vi "CanRxDetector.vi"() -> ()   [LabVIEW 2012]
panel:
  out "string":string
  in  "CAN_ID_Filter":u32 format="%08x"
  out "Picture":picture
  out "is active":bool
  out "error out":errorcluster {"code" format="%.0x"}
  out "Channel Status":T1 {"TX Load (%)" max=100 scale=0.0..100.0; "RX Load (%)" max=100 scale=0.0..100.0; "Line Status"."BUS Timing"."BTR1" format="%02x"; "Line Status"."BUS Timing"."BTR0" format="%02x"; "Line Status"."BUS Load (%)" max=100 step=1 scale=0.0..100.0}
  in  "Stop":bool
  out "Message Count":u32
  out "CAN message":T2 {"Data"."[4]" format="%02x"; "Data"."[7]" format="%02x"; "Data"."[6]" format="%02x"; "Data"."[5]" format="%02x"; "Data"."[3]" format="%02x"; "Data"."[2]" format="%02x"; "Data"."[1]" format="%02x"; "Data"."[0]" format="%02x"; "Timestamp" format="%08x"; "Arbitration ID" format="%08x"}
  out "IsRunning":bool
  # "CAN messages Log"
  # "CAN ID"
  # "CAN message"
  # "Channel Status"
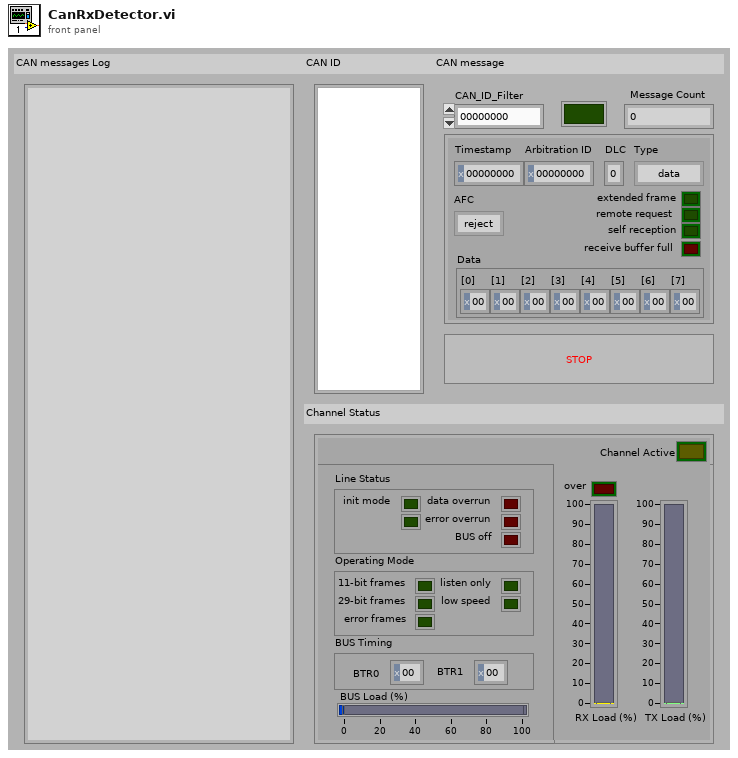
[diagram p1: front panel]
types:
  T1 = cluster{"Line Status":cluster{"Line Status":cluster{"init mode":bool, "TX pending":bool, "data overrun":bool, "error overrun":bool, "BUS off":bool}, "Operating Mode":cluster{"11-bit frames":bool, "29-bit frames":bool, "error frames":bool, "listen only":bool, "low speed":bool}, "BUS Timing":cluster{"BTR0":u8, "BTR1":u8}, "BUS Load (%)":u8}, "Channel Active":bool, "over":bool, "RX Load (%)":u8, "TX Load (%)":u8}
  T2 = cluster{"Timestamp":u32, "Arbitration ID":u32, "DLC":u8, "Type":enum8{"data", "info", "error", "status", "wakeup", "timer ovr", "timer reset"}, "AFC":enum8{"reject", "always", "filter 1", "filter 2"}, "extended frame":bool, "remote request":bool, "self reception":bool, "receive buffer full":bool, "Data":cluster{"[0]":u8, "[1]":u8, "[2]":u8, "[3]":u8, "[4]":u8, "[5]":u8, "[6]":u8, "[7]":u8}}
  T3 = cluster{"Width":u16, "Style":enum32{"Solid", "Dash", "Dot", "DashDot", "DashDotDot"}}
  T4 = cluster{"[0]":u8, "[1]":u8, "[2]":u8, "[3]":u8, "[4]":u8, "[5]":u8, "[6]":u8, "[7]":u8}
  T5 = cluster{"Data[0]":u8, "Data[1]":u8, "Data[2]":u8, "Data[3]":u8, "Data[4]":u8, "Data[5]":u8, "Data[6]":u8, "Data[7]":u8}
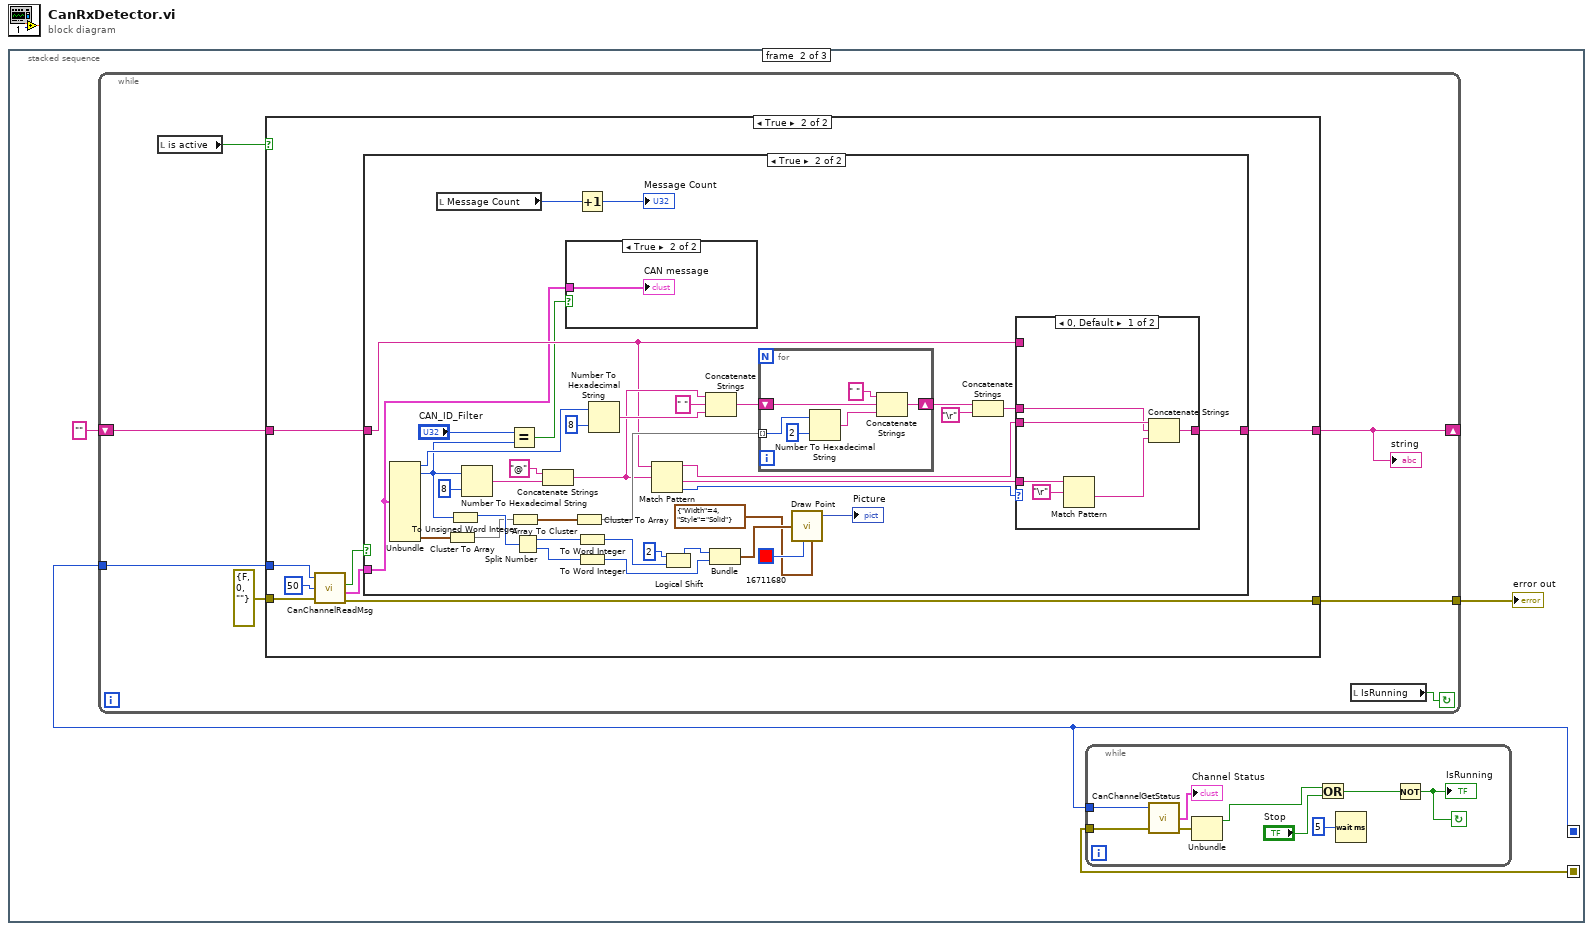
[diagram p0: block diagram]
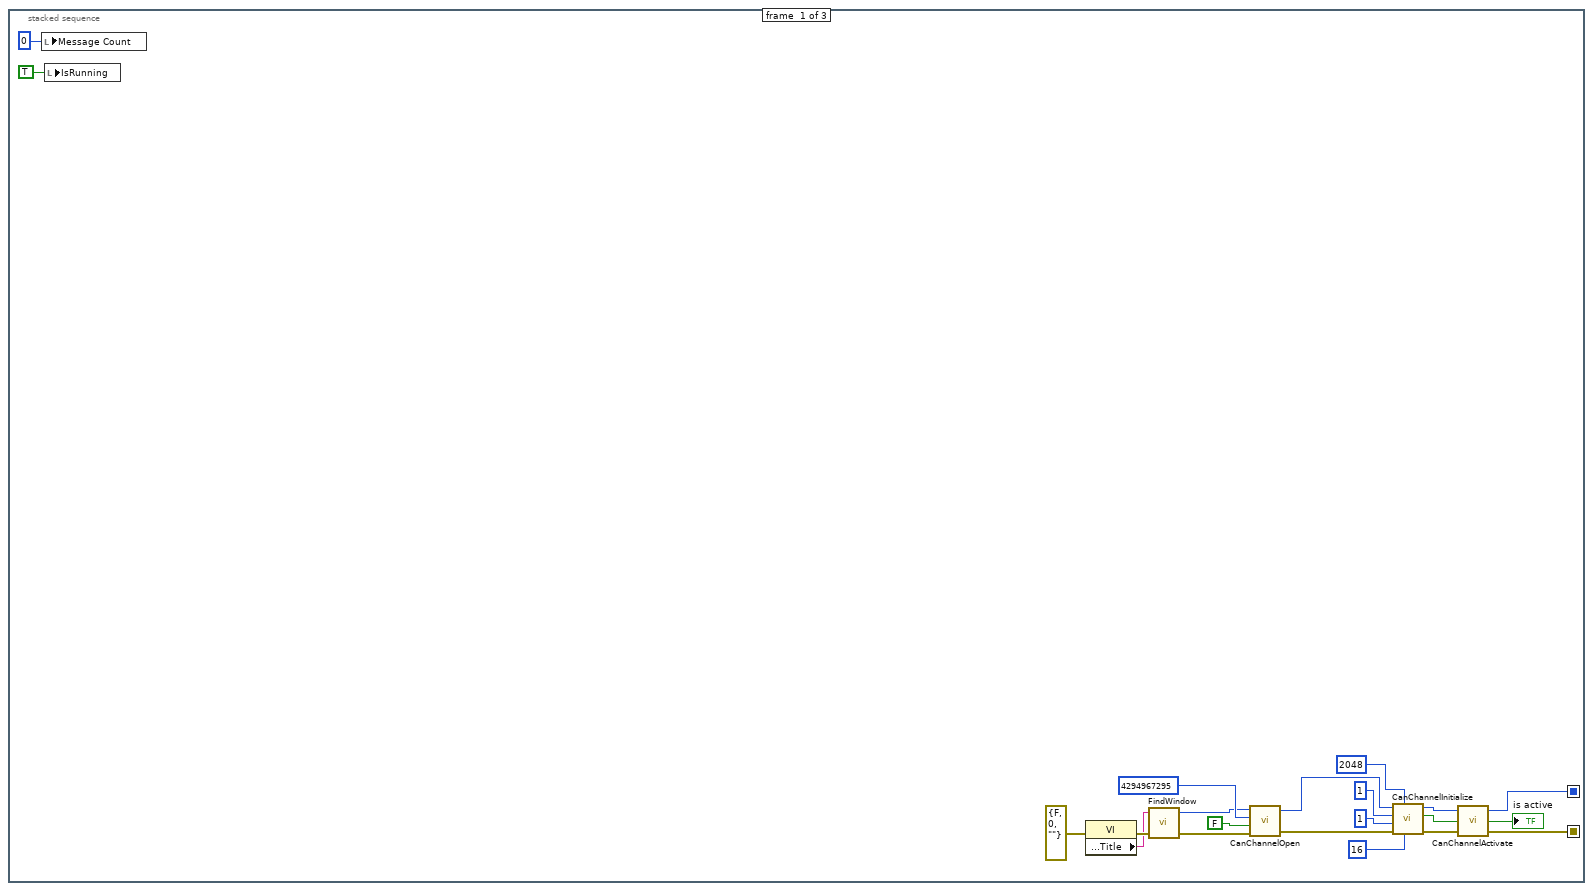
[diagram p2: hidden frame]
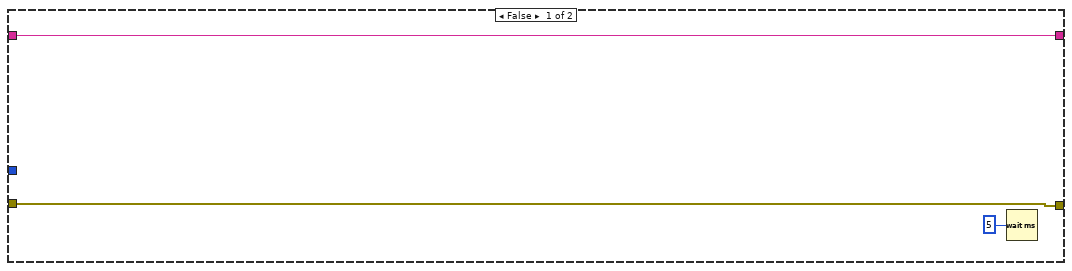
[diagram p3: hidden frame]
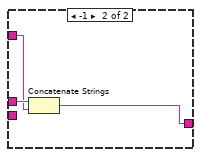
[diagram p6: hidden frame]
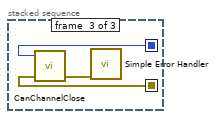
[diagram p7: hidden frame]
diagram:
  n1 = stacked-sequence {
    seq-local: [w2 _ _] -> [_ w24 w110]
    seq-local: [w3 _ _] -> [_ w25 w108]
    frame #0 {
      n2 = local write "Message Count"(u32 0 ("Message Count")) -> ()
      n3 = local write "IsRunning"(TRUE ("IsRunning")) -> ()
      n4 = property class="VI"(error in=errorcluster {"status"=FALSE, "code"=0, "source"=""}) -> (error out=w10:errorcluster, "Front Panel Window:Title"=w9:string)  [unwired: 1 in, 1 out]
      n5 = call "FindWindow.vi"("error in"=w10, "Window Title"=w9) -> ("error out"=w11:errorcluster, "HWND"=w12:u32)  [unwired: 2 in]
      n6 = call "CanChannelOpen.vi"("error in"=w11, "Exclusive"=FALSE, "CAN Number"=u32 4294967295, "Device Handle"=w12) -> ("error out"=w20:errorcluster, "CAN Channel Handle"=w19:u32)  [unwired: 1 in]
      n7 = call "CanChannelInitialize.vi"("TX Fifo Size"=u16 16 ("TX FIFO Size"), "RX Fifo Size"=u16 2048 ("RX FIFO Size"), "error in"=w20, "TX Threshold"=u16 1, "RX Threshold"=u16 1, "CAN Channel Handle in"=w19) -> ("error out"=w5:errorcluster, "Init OK"=w4:bool, "CAN Channel Handle out"=w6:u32)  [unwired: 1 in]
      n8 = call "CanChannelActivate.vi"("error in"=w5, "activate"=w4, "CAN Channel Handle in"=w6) -> ("error out"=w3:errorcluster, "is active"=→"is active":bool, "CAN Channel Handle out"=w2:u32)
    }
    frame #1 {
      n9 = while {
        tunnel: w24 -> [w31]
        tunnel: [w29] -> w23
        shift-right: [w27] -> _
        shift-left: "" ("string") -> [w26]
        stop <- w32 continue-if-true
        n10 = local read "is active"() -> (w30:bool)
        n11 = case shown="True" w30 {
          tunnel: w31 -> [_ w42]
          tunnel: [w34 w39] -> w29
          tunnel: errorcluster {"status"=FALSE, "code"=0, "source"=""} ("error in") -> [w34 w38]
          tunnel: [w33 w37] -> w27
          tunnel: w26 -> [w33 w36]
          frame False {
            n12 = Wait (ms)(milliseconds to wait=u32 5) -> ()  [unwired: 1 out]
          }
          frame True {
            n13 = call "CanChannelReadMsg.vi"("CAN Channel Handle in"=w42, "Milliseconds"=u32 50, "error in"=w38) -> ("Is Valid Message"=w41:bool, "CAN message"=w40:T2, "error out"=w39:errorcluster)  [unwired: 1 out]
            n14 = case shown="True" w41 {
              tunnel: w40 -> [_ w49]
              tunnel: [w44 w53] -> w37
              tunnel: w36 -> [w44 w54]
              frame False {
              }
              frame True {
                n15 = Unbundle(w49) -> ("Timestamp"=w64:u32, "Arbitration ID"=w47:u32, "Data"=w71:T4)  [unwired: 7 out]
                n16 = local read "Message Count"() -> (w82:u32)
                n17 = Cluster To Array(cluster=w71) -> (array=w70:u8[])
                n18 = To Unsigned Word Integer(number=w47) -> (unsigned 16bit integer=w74:u16)
                n19 = Number To Hexadecimal String(1:i16 8 ("width (-)"), 2:w47) -> (0:w59:string)
                n20 = Equal?(x="CAN_ID_Filter", y=w47) -> (x = y?=w50:bool)
                n21 = Array To Cluster(array=w70) -> (cluster=w69:T5)
                n22 = Split Number(x=w74) -> (hi(x)=w79:u8, lo(x)=w78:u8)
                n23 = Concatenate Strings("@" ("string"), w59) -> (w58:string)
                n24 = case shown="True" w50 {
                  tunnel: w49 -> [_ w83]
                  frame False {
                  }
                  frame True {
                    "CAN message" <- w83
                  }
                }
                n25 = Cluster To Array(cluster=w69) -> (array=w68:u8[])
                n26 = Increment(x=w82) -> (x+1=→"Message Count":u32)
                n27 = To Word Integer(number=w79) -> (16bit integer=w72:i16)
                n28 = To Word Integer(number=w78) -> (16bit integer=w46:i16)
                n29 = Number To Hexadecimal String(1:i16 8 ("width (-)"), 2:w64) -> (0:w63:string)
                n30 = Match Pattern(string=w54, regular expression=w58) -> (before substring=w52:string, after substring=w51:string, offset past match=w56:i32)  [unwired: 1 in, 1 out]
                n31 = Logical Shift(y=i16 2, x=w72) -> (x << y=w45:i16)
                n32 = Concatenate Strings(w58, " " ("string"), w63) -> (w62:string)
                n33 = Bundle(w45, w46) -> (w80:cluster{i16, i16})  [unwired: 1 in]
                n34 = for {
                  tunnel: w68 -> [w98] mode=indexing
                  shift-right: [w94] -> w61
                  shift-left: w62 -> [w95]
                  n35 = Number To Hexadecimal String(1:i16 2 ("width (-)"), 2:w98) -> (0:w96:string)
                  n36 = Concatenate Strings(" " ("string"), w95, w96) -> (w94:string)
                }
                n37 = call <vilib>:"Draw Point.vi"("point(x,y)"=w80, "color(black)"=u32 16711680, "pen"=T3 {"Width"=4, "Style"=enum."Solid"}) -> ("new picture"=→"Picture":picture)  [unwired: 6 in]
                n38 = Concatenate Strings(w61, "\r") -> (w55:string)
                n39 = case shown="0, Default" w56 {
                  tunnel: w55 -> [w88 w92]
                  tunnel: w54 -> [_ w91]
                  tunnel: [w84 w90] -> w53
                  tunnel: w52 -> [w89 _]
                  tunnel: w51 -> [w87 _]
                  frame 0, Default {
                    n40 = Match Pattern(string=w87, regular expression="\r") -> (after substring=w85:string)  [unwired: 1 in, 3 out]
                    n41 = Concatenate Strings(w89, w88, w85) -> (w84:string)
                  }
                  frame -1 {
                    n42 = Concatenate Strings(w92, w91) -> (w90:string)
                  }
                }
              }
            }
          }
        }
        "string" <- w27
        n43 = local read "IsRunning"() -> (w32:bool)
      }
      "error out" <- w23
      n44 = while {
        tunnel: w24 -> [w99]
        tunnel: w25 -> [w100]
        stop <- w101 continue-if-true
        n45 = call "CanChannelGetStatus.vi"("error in"=w100, "CAN Channel Handle in"=w99) -> ("error out"=w106:errorcluster, "Channel Status"=→"Channel Status":T1)  [unwired: 1 in, 1 out]
        n46 = Unbundle(w106) -> ("status"=w105:bool)  [unwired: 2 out]
        n47 = Or(x=w105, y="Stop") -> (x .or. y?=w104:bool)
        n48 = Wait (ms)(milliseconds to wait=u32 5) -> ()  [unwired: 1 out]
        n49 = Not(x=w104) -> (.not. x?=w101:bool)
        "IsRunning" <- w101
      }
    }
    frame #2 {
      n50 = call "CanChannelClose.vi"("error in"=w108, "CAN Channel Handle"=w110) -> ("error out"=w109:errorcluster)  [unwired: 3 in]
      n51 = call <vilib>:"Simple Error Handler.vi"("error in (no error)"=w109) -> ()  [unwired: 4 in, 5 out]
    }
  }
